vi "ErrorCheckHWI.vi"(8 "error in (no error)":errorcluster, 11 "Pulseblaster in":refnum<class "Pulseblaster.lvclass">) -> (0 "error out":errorcluster, 3 "Pulseblaster out":refnum<class "Pulseblaster.lvclass">)   [LabVIEW 2013, in "Pulseblaster.lvclass"]
uses:
  Pulseblaster.lvclass
  Pulseblaster.lvclass/Pulseblaster.ctl
  Globals/Total Time.vi
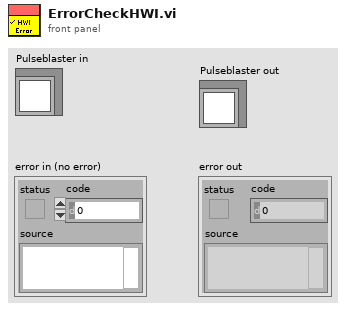
[diagram p1: front panel]
types:
  T1 = cluster{"Output Bits":u32, "Data Field":u32, "OP Code":u8, "Delay Count":u64}[]
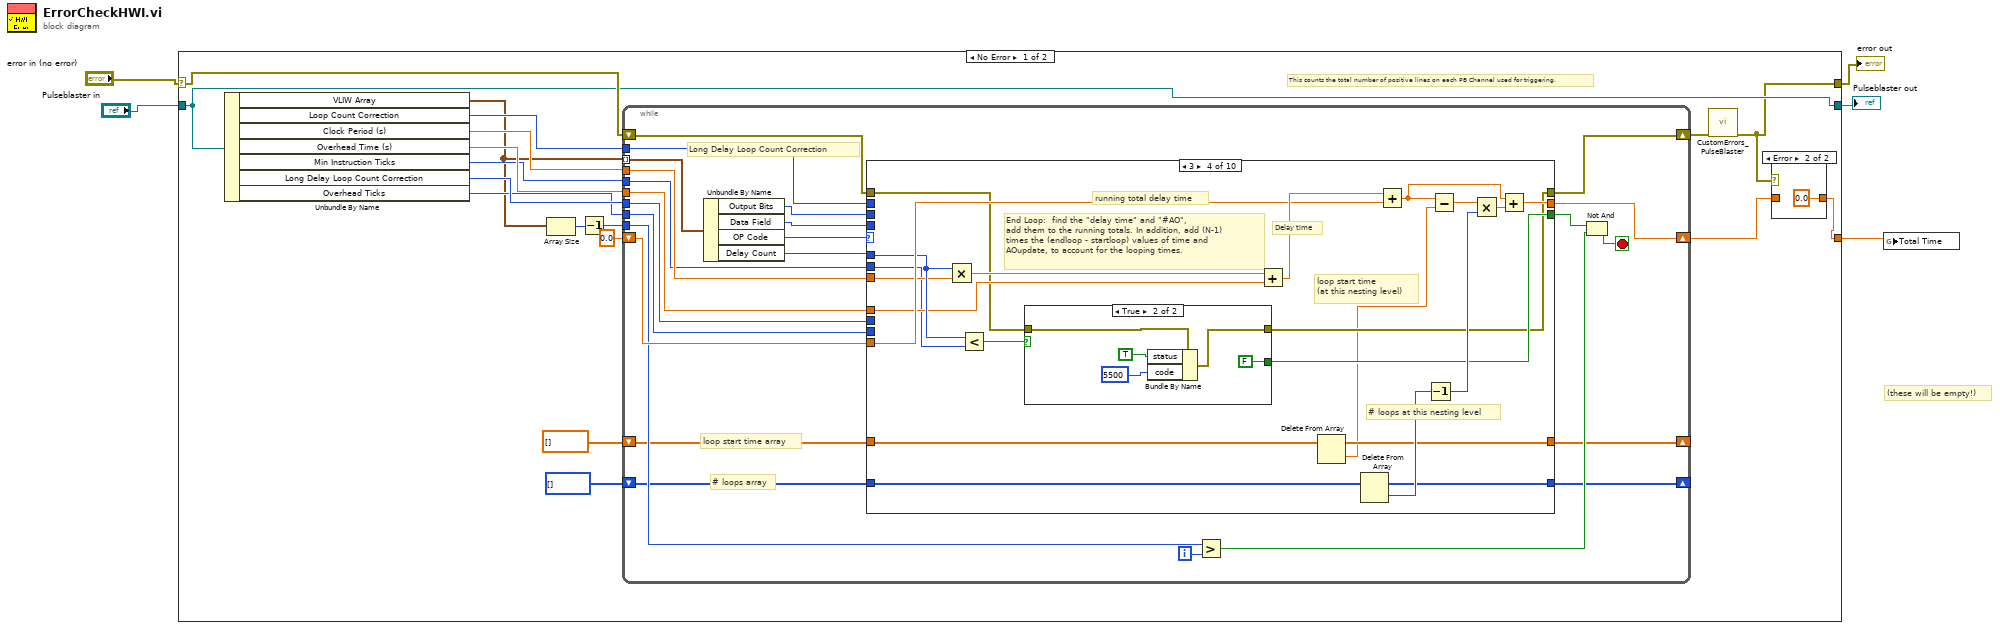
[diagram p0: block diagram]
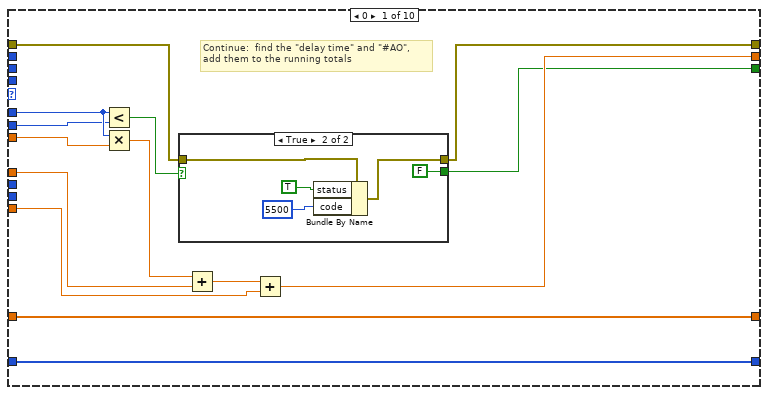
[diagram p3: hidden frame]
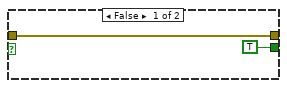
[diagram p4: hidden frame]
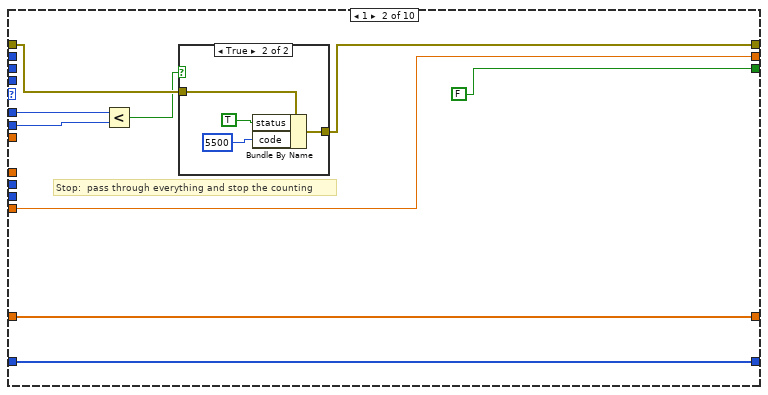
[diagram p5: hidden frame]
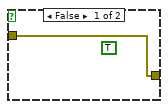
[diagram p6: hidden frame]
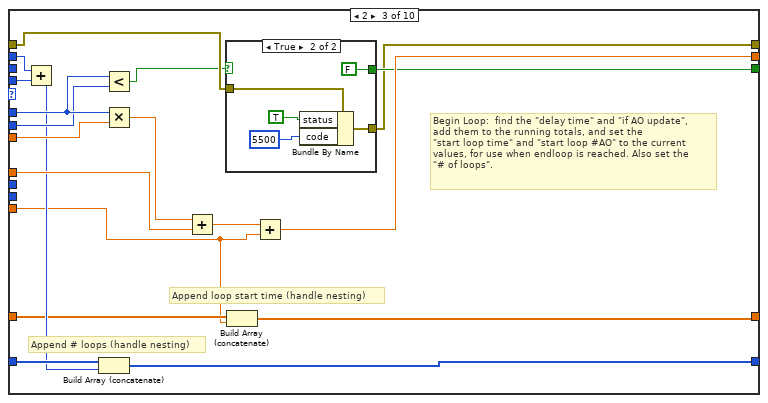
[diagram p7: hidden frame]
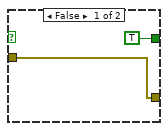
[diagram p8: hidden frame]
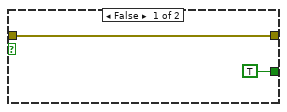
[diagram p9: hidden frame]
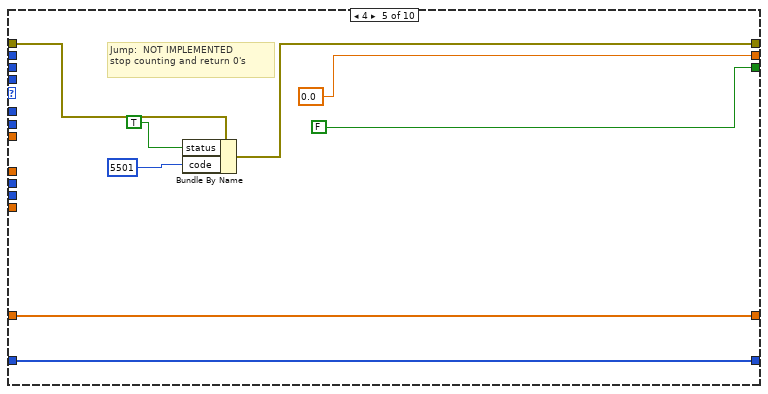
[diagram p10: hidden frame]
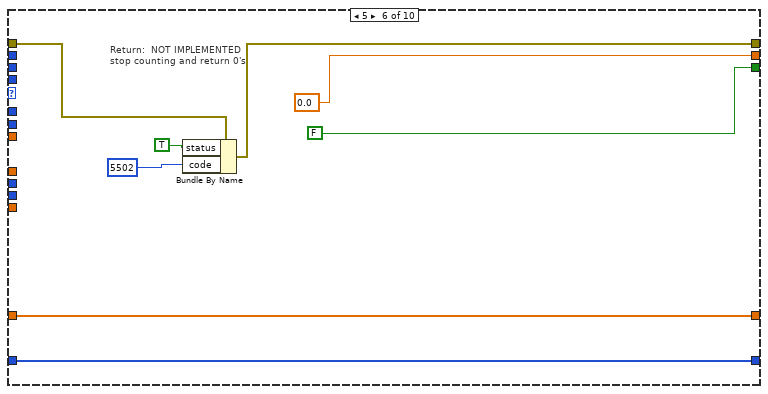
[diagram p11: hidden frame]
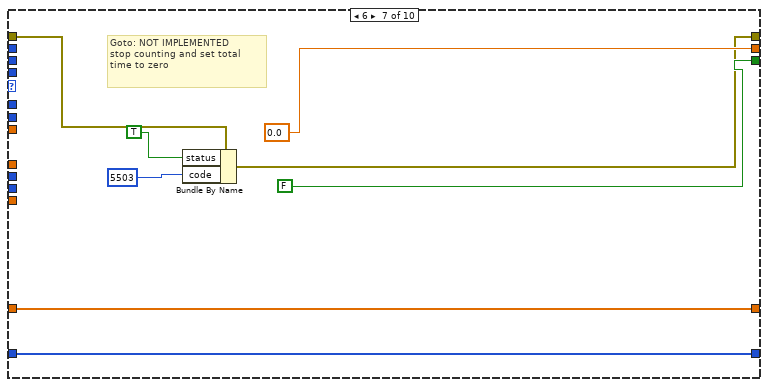
[diagram p12: hidden frame]
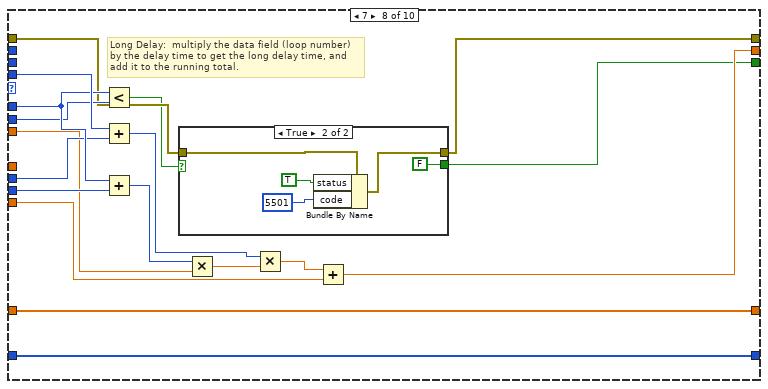
[diagram p13: hidden frame]
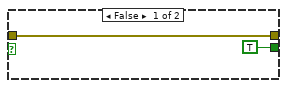
[diagram p14: hidden frame]
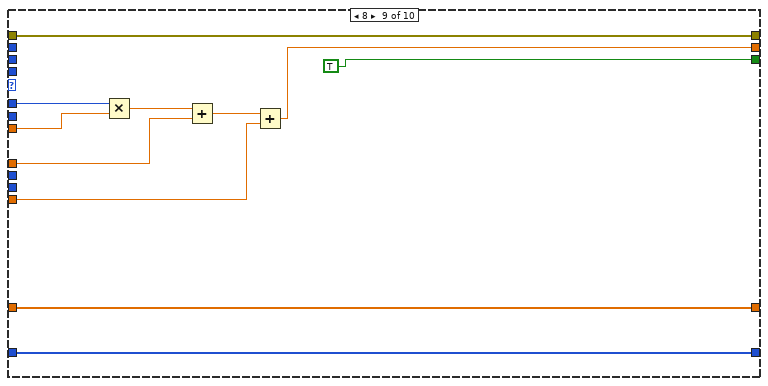
[diagram p15: hidden frame]
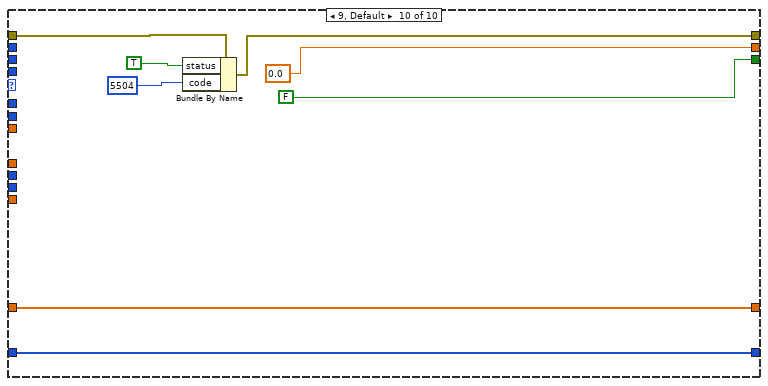
[diagram p16: hidden frame]
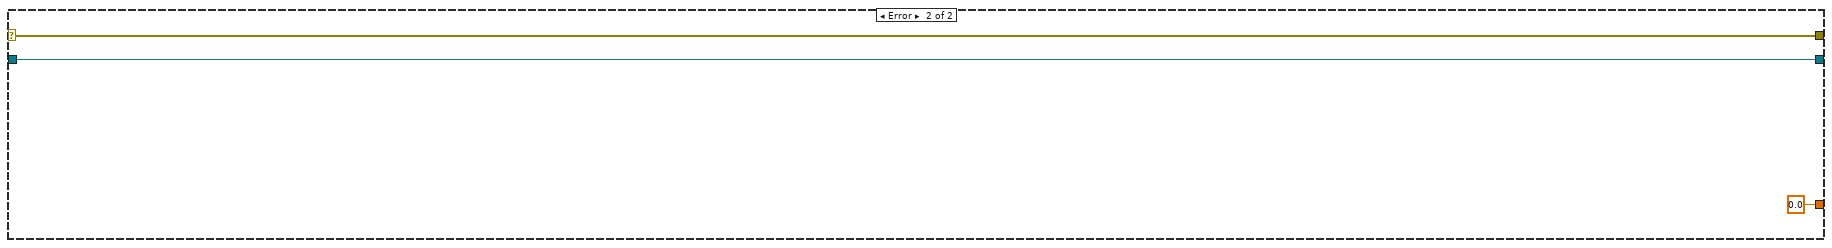
[diagram p17: hidden frame]
diagram:
  # "(these will be empty!)"
  n1 = case shown="No Error" "error in (no error)" {
    selector: "error in (no error)" -> [w21 w210]
    tunnel: [w11 w210] -> w3
    tunnel: "Pulseblaster in" -> [w12 w208]
    tunnel: [w12 w208] -> w2
    tunnel: [w9 0.0 ("Start loop time")] -> w1
    frame No Error {
      # "This counts the total number of positive lines on each PB Channel used for triggering."
      n2 = Unbundle By Name(w12) -> ("VLIW Array"=w14:T1, "Loop Count Correction"=w20:u8, "Clock Period (s)"=w19:dbl, "Overhead Time (s)"=w18:dbl, "Min Instruction Ticks"=w17:u8, "Long Delay Loop Count Correction"=w16:u8, "Overhead Ticks"=w15:u8)
      n3 = Array Size(array=w14) -> (size(s)=w23:i32)
      n4 = Decrement(x=w23) -> (x-1=w22:i32)
      n5 = while {
        tunnel: w22 -> [w36]
        shift-left: 0.0 -> [w48]
        shift-right: [w47] -> w10
        tunnel: w14 -> [w49] mode=indexing
        tunnel: w20 -> [w35]
        tunnel: w19 -> [w34]
        tunnel: w18 -> [w33]
        tunnel: w17 -> [w32]
        tunnel: w16 -> [w31]
        tunnel: w15 -> [w30]
        shift-right: [w41] -> w13
        shift-left: w21 -> [w42]
        shift-right: [w28] -> _
        shift-left: u32[] [] ("# loops Array") -> [w29]
        shift-right: [w27] -> _
        shift-left: dbl[] [] ("Start Loop Time Array") -> [w26]
        i -> [w37]
        stop <- w39 stop-if-true
        # "loop start time array"
        # "# loops array"
        # "Long Delay Loop Count Correction"
        n6 = Unbundle By Name(w49) -> ("Output Bits"=w44:u32, "Data Field"=w43:u32, "OP Code"=w45:u8, "Delay Count"=w46:u64)
        n7 = case shown="3" w45 {
          tunnel: w46 -> [w59 w78 w100 w125 _ _ _ w174 w194 _]
          tunnel: w44 -> [_ _ _ _ _ _ _ _ _ _]
          tunnel: w48 -> [w61 w79 w85 w126 _ _ _ w175 w195 _]
          tunnel: [w62 w79 w101 w127 0.0 0.0 0.0 w179 w193 0.0] -> w47
          tunnel: [w53 FALSE w94 w118 FALSE FALSE FALSE w166 TRUE FALSE] -> w40
          tunnel: w43 -> [_ _ w91 _ _ _ _ w181 _ _]
          tunnel: w42 -> [w55 w75 w96 w120 w143 w152 w161 w169 w198 w205]
          tunnel: [w52 w73 w93 w117 w142 w151 w160 w167 w198 w204] -> w41
          tunnel: w35 -> [_ _ w92 _ _ _ _ _ _ _]
          tunnel: w34 -> [w58 _ w99 w123 _ _ _ w171 w192 _]
          tunnel: w33 -> [w57 _ w98 w122 _ _ _ _ w191 _]
          tunnel: w32 -> [w56 w76 w97 w121 _ _ _ w170 _ _]
          tunnel: w31 -> [_ _ _ _ _ _ _ w173 _ _]
          tunnel: w30 -> [_ _ _ _ _ _ _ w172 _ _]
          tunnel: w29 -> [w51 w72 w90 w116 w141 w149 w157 w165 w190 w201]
          tunnel: [w51 w72 w89 w114 w141 w149 w157 w165 w190 w201] -> w28
          tunnel: [w50 w71 w86 w112 w140 w148 w156 w164 w189 w200] -> w27
          tunnel: w26 -> [w50 w71 w87 w113 w140 w148 w156 w164 w189 w200]
          frame 0 {
            # "Continue:  find the \"delay time\" and \"#AO\",\nadd them to the running totals"
            n8 = Less?(x=w59, y=w56) -> (x < y?=w54:bool)
            n9 = Multiply(x=w59, y=w58) -> (x*y=w63:dbl)
            n10 = case shown="True" w54 {
              tunnel: w55 -> [w65 w70]
              tunnel: [w65 w68] -> w52
              tunnel: [TRUE FALSE] -> w53
              frame False {
              }
              frame True {
                n11 = Bundle By Name(cluster=w70, "status"=TRUE, "code"=5500) -> (w68:errorcluster)
              }
            }
            n12 = Add(x=w63, y=w57) -> (x+y=w60:dbl)
            n13 = Add(x=w60, y=w61) -> (x+y=w62:dbl)
          }
          frame 1 {
            # "Stop:  pass through everything and stop the counting"
            n14 = Less?(x=w78, y=w76) -> (x < y?=w74:bool)
            n15 = case shown="True" w74 {
              tunnel: w75 -> [w80 w84]
              tunnel: [w80 w82] -> w73
              frame False {
                (unwired) TRUE
              }
              frame True {
                n16 = Bundle By Name(cluster=w84, "status"=TRUE, "code"=5500) -> (w82:errorcluster)
              }
            }
          }
          frame 2 {
            # "Append loop start time (handle nesting)"
            # "Append # loops (handle nesting)"
            # "Begin Loop:  find the \"delay time\" and \"if AO update\",\nadd them to the running totals, and set the \n\"start loop time\" and \"start loop #AO\" to the current\nvalues, for use when endloop is reached. Also set the\n\"# of loops\"."
            n17 = Add(x=w92, y=w91) -> (x+y=w88:u32)
            n18 = Build Array (concatenate)(w90, w88) -> (w89:u32[])
            n19 = Less?(x=w100, y=w97) -> (x < y?=w95:bool)
            n20 = Multiply(x=w100, y=w99) -> (x*y=w103:dbl)
            n21 = Add(x=w103, y=w98) -> (x+y=w102:dbl)
            n22 = case shown="True" w95 {
              tunnel: w96 -> [w105 w110]
              tunnel: [w105 w108] -> w93
              tunnel: [TRUE FALSE] -> w94
              frame False {
              }
              frame True {
                n23 = Bundle By Name(cluster=w110, "status"=TRUE, "code"=5500) -> (w108:errorcluster)
              }
            }
            n24 = Build Array (concatenate)(w87, w85) -> (w86:dbl[])
            n25 = Add(x=w102, y=w85) -> (x+y=w101:dbl)
          }
          frame 3 {
            # "loop start time\n(at this nesting level)"
            # "# loops at this nesting level"
            # "running total delay time"
            # "Delay time"
            # "End Loop:  find the \"delay time\" and \"#AO\",\nadd them to the running totals. In addition, add (N-1)\ntimes the (endloop - startloop) values of time and\nAOupdate, to account for the looping times."
            n26 = Multiply(x=w125, y=w123) -> (x*y=w132:dbl)
            n27 = Less?(x=w125, y=w121) -> (x < y?=w119:bool)
            n28 = case shown="True" w119 {
              tunnel: w120 -> [w134 w139]
              tunnel: [w134 w137] -> w117
              tunnel: [TRUE FALSE] -> w118
              frame False {
              }
              frame True {
                n29 = Bundle By Name(cluster=w139, "status"=TRUE, "code"=5500) -> (w137:errorcluster)
              }
            }
            n30 = Add(x=w132, y=w122) -> (x+y=w131:dbl)
            n31 = Delete From Array(array=w113) -> (deleted portion=w111:dbl, array with subset deleted=w112:dbl[])  [unwired: 2 in]
            n32 = Delete From Array(array=w116) -> (deleted portion=w115:u32, array with subset deleted=w114:u32[])  [unwired: 2 in]
            n33 = Add(x=w131, y=w126) -> (x+y=w128:dbl)
            n34 = Decrement(x=w115) -> (x-1=w124:u32)
            n35 = Subtract(x=w128, y=w111) -> (x-y=w130:dbl)
            n36 = Multiply(x=w130, y=w124) -> (x*y=w129:dbl)
            n37 = Add(x=w128, y=w129) -> (x+y=w127:dbl)
          }
          frame 4 {
            # "Jump:  NOT IMPLEMENTED\nstop counting and return 0's"
            n38 = Bundle By Name(cluster=w143, "status"=TRUE, "code"=5501) -> (w142:errorcluster)
          }
          frame 5 {
            # "Return:  NOT IMPLEMENTED\nstop counting and return 0's"
            n39 = Bundle By Name(cluster=w152, "status"=TRUE, "code"=5502) -> (w151:errorcluster)
          }
          frame 6 {
            # "Goto: NOT IMPLEMENTED\nstop counting and set total\ntime to zero"
            n40 = Bundle By Name(cluster=w161, "status"=TRUE, "code"=5503) -> (w160:errorcluster)
          }
          frame 7 {
            # "Long Delay:  multiply the data field (loop number)\nby the delay time to get the long delay time, and\nadd it to the running total."
            n41 = Less?(x=w174, y=w170) -> (x < y?=w168:bool)
            n42 = Add(x=w181, y=w173) -> (x+y=w176:u32)
            n43 = Add(x=w174, y=w172) -> (x+y=w180:u64)
            n44 = case shown="True" w168 {
              tunnel: w169 -> [w183 w188]
              tunnel: [w183 w186] -> w167
              tunnel: [TRUE FALSE] -> w166
              frame False {
              }
              frame True {
                n45 = Bundle By Name(cluster=w188, "status"=TRUE, "code"=5501) -> (w186:errorcluster)
              }
            }
            n46 = Multiply(x=w180, y=w171) -> (x*y=w177:dbl)
            n47 = Multiply(x=w176, y=w177) -> (x*y=w178:dbl)
            n48 = Add(x=w178, y=w175) -> (x+y=w179:dbl)
          }
          frame 8 {
            n49 = Multiply(x=w194, y=w192) -> (x*y=w197:dbl)
            n50 = Add(x=w197, y=w191) -> (x+y=w196:dbl)
            n51 = Add(x=w196, y=w195) -> (x+y=w193:dbl)
          }
          frame 9, Default {
            n52 = Bundle By Name(cluster=w205, "status"=TRUE, "code"=5504) -> (w204:errorcluster)
          }
        }
        n53 = Greater?(x=w36, y=w37) -> (0:w38:bool)
        n54 = Not And(1:w38, 2:w40) -> (0:w39:bool)
      }
      n55 = call "CustomErrors_PulseBlaster.vi"("error in (no error)"=w13) -> ("error out"=w11:errorcluster)  [unwired: 10 in]
      n56 = case shown="Error" w11 {
        tunnel: w10 -> [w24 _]
        tunnel: [w24 0.0 ("Start loop time")] -> w9
        frame No Error {
        }
        frame Error {
        }
      }
    }
    frame Error {
    }
  }
  "error out" <- w3
  "Pulseblaster out" <- w2
  n57 = global write "Total Time.vi" "Total Time"(w1) -> ()
